vi "Continuous Analog Output Non Regeneration DAQ.vi"() -> ()   [LabVIEW 2020]
uses:
  <resource>/objmgr/daqmx.rc
  <vilib>/DAQmx/create/channels.llb/DAQmx Create Channel (AO-Voltage-Basic).vi
  <vilib>/DAQmx/configure/timing.llb/DAQmx Timing (Sample Clock).vi
  <vilib>/DAQmx/write.llb/DAQmx Write (Analog 1D DBL 1Chan NSamp).vi
panel:
  in  "Stop":bool
  in  "Frequency":dbl(slide)=10.1 scale=0.0..10.0
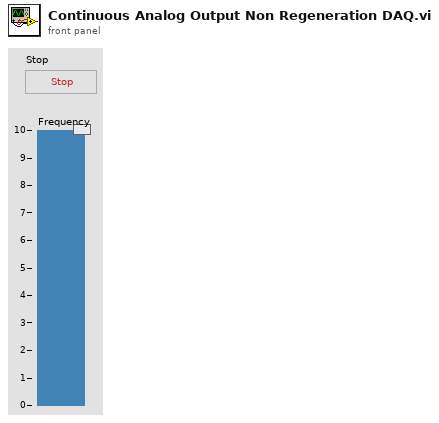
[diagram p1: front panel]
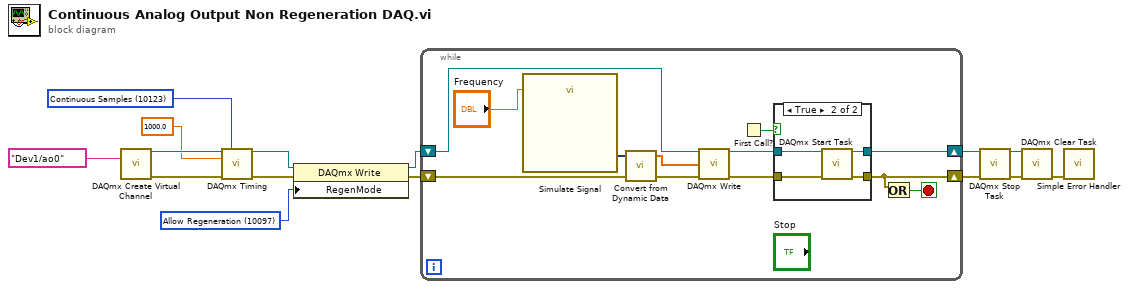
[diagram p0: block diagram]
diagram:
  w3 = 10097 items=["Allow Regeneration"=10097, "Do Not Allow Regeneration"=10158] ("RegenMode")
  w11 = 10123 items=["Finite Samples"=10178, "Continuous Samples"=10123, "Hardware Timed Single Point"=12522] ("sample mode")
  n1 = call-poly <vilib>:"DAQmx Create Virtual Channel.vi"("physical channels"=tag "Dev1/ao0") -> ("task out"=w14:refnum<k21>, "error out"=w13:errorcluster)  [unwired: 13 in]
  n2 = call-poly <vilib>:"DAQmx Timing.vi"("task/channels in"=w14, "sample mode"=w11, "rate"=1000.0, "error in"=w13) -> ("task out"=w7:refnum<k21>, "error out"=w6:errorcluster)  [unwired: 10 in]
  n3 = property class="DAQmx Write"(reference=w7, error in=w6, "RegenMode"=w3) -> (reference out=w5:refnum<k21>, error out=w4:errorcluster)
  n4 = while {
    shift-right: [w20] -> w2
    shift-left: w5 -> [w22]
    shift-right: [w17] -> w1
    shift-left: w4 -> [w21]
    stop <- w18 stop-if-true
    n5 = call "Simulate Signal"("Frequency"="Frequency") -> ("Triangle"=w26:dynamicdata)  [unwired: 13 in, 1 out]
    n6 = call "Convert from Dynamic Data"("Dynamic Data Type"=w26) -> ("Array"=w25:dbl[])  [unwired: 3 in]
    n7 = call-poly <vilib>:"DAQmx Write.vi"("task/channels in"=w22, "data"=w25, "error in"=w21) -> ("task out"=w24:refnum<k21>, "error out"=w23:errorcluster)  [unwired: 10 in, 1 out]
    n8 = First Call?() -> (First Call?: T/F=w16:bool)
    n9 = case shown="True" w16 {
      tunnel: w24 -> [w28 w32]
      tunnel: w23 -> [w27 w31]
      tunnel: [w28 w30] -> w20
      tunnel: [w27 w29] -> w17
      frame False {
      }
      frame True {
        n10 = call <vilib>:"DAQmx Start Task.vi"("task/channels in"=w32, "error in"=w31) -> ("task out"=w30:refnum<k21>, "error out"=w29:errorcluster)  [unwired: 12 in]
      }
    }
    n11 = Or(x=w17) -> (x .or. y?=w18:bool)  [unwired: 1 in]
  }
  n12 = call <vilib>:"DAQmx Stop Task.vi"("task/channels in"=w2, "error in"=w1) -> ("task out"=w10:refnum<k21>, "error out"=w9:errorcluster)  [unwired: 12 in]
  n13 = call <vilib>:"DAQmx Clear Task.vi"("task in"=w10, "error in"=w9) -> ("error out"=w8:errorcluster)  [unwired: 13 in]
  n14 = call <vilib>:"Simple Error Handler.vi"("error in (no error)"=w8) -> ()  [unwired: 4 in, 5 out]
